vi "TB-Create Stimulus.vi"(0 "StimChan In":T24(xcontrol), 5 "state":T1, 11 "error in (no error)":errorcluster, 12 "Fine adjust (dB)":dbl) -> (4 "StimChan Out":T24(xcontrol), 6 "state out":T1, 8 "Stimulus":dbl[][](array[numeric]), 15 "error out":errorcluster)   [LabVIEW 2020]
uses:
  epl-vi-lib/Signal Synthesis VIs/Controls/Stimulus Channel XCtl/Stimulus Channel.xctl
  Typedefs/TB-Stimulus State.ctl
  <vilib>/sound2/lvsound2.llb/Sound File Refnum.ctl
  epl-vi-lib/Utility VIs/Math VIs/dB to Linear (scalar).vi
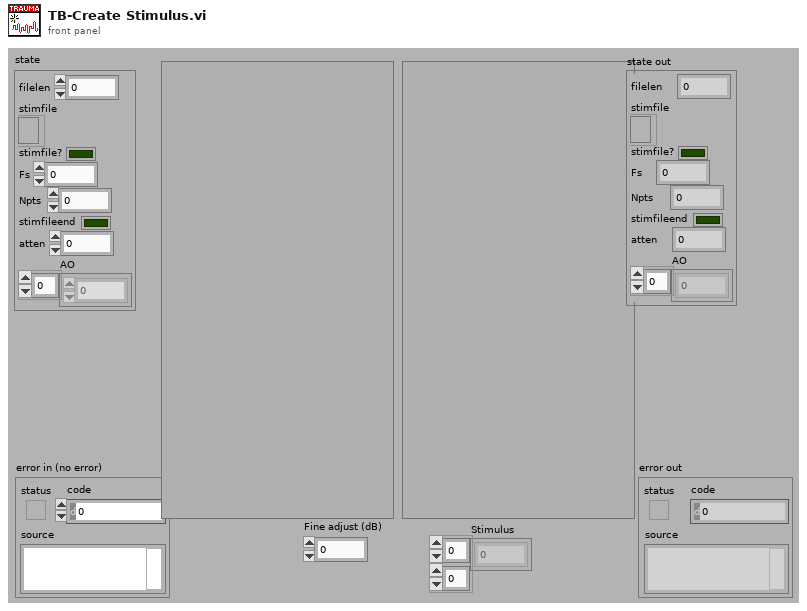
[diagram p1: front panel]
types:
  T1 = typedef "TB-Stimulus State.ctl" = cluster{"filelen":i32, "stimfile":T2, "stimfile?":bool, "Fs":dbl, "Npts":i32, "stimfileend":bool, "atten":dbl, "AO":i32[]}
  T2 = typedef "Sound File Refnum.ctl" = refnum<file>
  T3 = typedef "Waveform XCtl.xctl/Waveform Data.ctl" = cluster{"Type":T4, "Tone":T5, "Pulse Train":T6, "Noise":T9, "File":T10, "FMSweep":T11, "Chirp Train":T12, "Complex Tone":cluster{"Params":T14, "Data":T16}, "Moving Ripple":T17}
  T4 = typedef "Waveform Enum.ctl" = enum16{"OFF", "Tone", "Noise", "Pulse Train", "File", "FM Sweep", "Chirp Train", "Complex Tone", "FM Tone", "Moving Ripple"}
  T5 = typedef "Tone Params.ctl" = cluster{"Frequency (kHz)":dbl, "Last Freq":dbl, "Last Phase":dbl}
  T6 = typedef "Pulse Train Params.ctl" = cluster{"Pulse width (us)":dbl, "Pulse rate (Hz)":dbl, "Gap (ms)":dbl, "Polarity":T7, "PT State":T8, "Asynch":bool}
  T7 = typedef "Pulse Polarity.ctl" = enum16{"POS", "NEG", "POS-NEG", "NEG-POS"}
  T8 = typedef "PT-Continuous State.ctl" = cluster{"Template":dbl[], "Nperiod":i32, "Index":i32, "Pulse Rate (Hz)":dbl, "Phase (cycles)":dbl, "Noff":i32}
  T9 = typedef "Noise Params.ctl" = cluster{"InvFilt":bool, "Noise":dbl[], "CurPt":i32, "Aweight":bool, "Seed":i32, "afile":path}
  T10 = typedef "StimFile-Params.ctl" = cluster{"Filename":path, "Signal":dbl[], "Channel":i32, "stream":bool, "offset":i32, "nreps":i32, "loops":i32, "Randomize":bool, "order":i32[], "Seed":i32, "Tokens":i32}
  T11 = typedef "FM Sweep Params.ctl" = cluster{"Rate (oct/s)":dbl, "Fmin (Hz)":dbl, "Fmax (Hz)":dbl, "Ramp (ms)":dbl, "Linear":bool}
  T12 = typedef "Chirp Train.ctl" = cluster{"Params":T13, "Data":cluster{"WF":dbl[]}}
  T13 = typedef "Chirp Train Params.ctl" = cluster{"Fmin (kHz)":dbl, "Fmax (kHz)":dbl, "Compensate":bool, "Duration (ms)":dbl}
  T14 = typedef "CT-Params.ctl" = cluster{"F0 (Hz)":dbl, "Band":cluster{"Flow (Hz)":dbl, "Fhigh (Hz)":dbl}, "Phase":T15, "Min F0 (Hz)":dbl, "Max F0 (Hz)":dbl, "ContinRandPhase":bool, "Max peak factor":dbl, "Max mod depth":dbl, "MinHarmNum":i32, "MaxHarmNum":i32, "Level Mode":enum16{"per component", "overall rms"}, "% jitter":dbl}
  T15 = typedef "CT-Phase Enum.ctl" = enum16{"Cosine", "Random", "Alternating"}
  T16 = typedef "CT-Runtime Data.ctl" = cluster{"Ncomp":i32, "MinHarm":i32, "Phase":dbl[], "Amplitude":dbl[], "Npts/frame":i32, "Last F0":dbl, "Fmin":dbl, "Fmax":dbl, "Lslope":dbl, "randphase":bool, "overall rms":bool, "fmult":dbl[], "jittered":bool}
  T17 = typedef "Moving Ripple.ctl" = cluster{"Params":T18, "Data":T19}
  T18 = typedef "Moving Ripple.Params.ctl" = cluster{"Fmin":dbl, "Fmax":dbl, "Density":dbl, "Velocity":dbl, "Depth":dbl, "Phase":dbl, "Comp/oct":i32}
  T19 = typedef "Moving Ripple.Data.ctl" = cluster{"Freq":dbl[], "A":dbl[], "phase":dbl[], "Phase":dbl}
  T20 = typedef "Filter XCtl.xctl/Filter Data.ctl" = cluster{"CF (kHz)":dbl, "BW (kHz)":dbl, "IIR Filter Cluster":cluster{"filter structure":enum32{"IIR 2nd Order", "IIR 4th Order"}, "Reverse Coefficients":dbl[], "Forward Coefficients":dbl[]}, "Final Filter State":dbl[], "Scale Factor":dbl, "Final Filter State 2":dbl[], "Quadrature":bool, "Type":enum16{"Lowpass", "Highpass", "Bandpass", "Bandstop", "OFF"}}
  T21 = typedef "Gate Control.xctl/Gate Data.ctl" = cluster{"Active":bool, "Delay (ms)":dbl, "Width (ms)":dbl, "Ramp (ms)":dbl}
  T22 = typedef "Level XCtl.xctl/Level Data.ctl" = cluster{"Level":dbl, "Units":T23, "Max":dbl, "Multiplier":dbl, "Cal File":path, "Cal":cluster{"Freq (Hz)":dbl[], "Mag (dB SPL)":dbl[], "Phase (deg)":dbl[]}}
  T23 = typedef "Level Units.ctl" = enum16{"dB atten", "dB SPL", "dB re 1 Vrms", "dB V/Hz½", "mW", "dB HL", "Volts", "dB mW"}
  T24 = cluster{"Waveform":T3, "Filter":T20, "Gate":T21, "Level":T22}
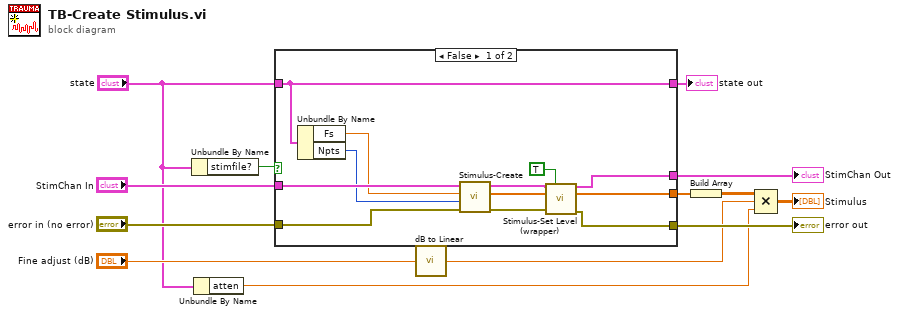
[diagram p0: block diagram]
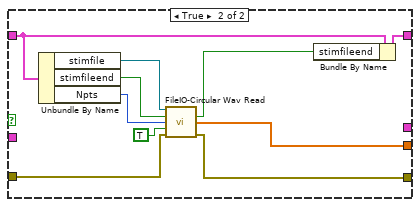
[diagram p2: hidden frame]
diagram:
  n1 = Unbundle By Name("state") -> ("stimfile?"=w4:bool)
  n2 = Unbundle By Name("state") -> ("atten"=w1:dbl)
  n3 = case shown="False" w4 {
    tunnel: "error in (no error)" -> [w25 w29]
    tunnel: "StimChan In" -> [w24 _]
    tunnel: [w19 _] -> w11
    tunnel: [w18 w27] -> w10
    tunnel: [w17 w28] -> w9
    tunnel: "state" -> [w14 w35]
    tunnel: [w14 w34] -> w3
    frame False {
      n4 = Unbundle By Name(w14) -> ("Fs"=w16:dbl, "Npts"=w15:i32)
      n5 = call "Stimulus-Create.vi"("error in (no error)"=w25, "Npts"=w15, "Sampling Rate (Hz)"=w16, "Stimulus Channel"=w24) -> ("error out"=w22:errorcluster, "Waveform"=w21:dbl[], "Stimulus Channel out"=w20:T24)  [unwired: 4 in, 1 out]
      n6 = call "Stimulus-Set Level (wrapper).vi"("Stimulus Channel"=w20, "Apply multiplier? (F)"=TRUE ("Apply multiplier?"), "Waveform in"=w21, "error in (no error)"=w22) -> ("Stimulus Channel out"=w19:T24, "Waveform out"=w18:dbl[], "error out"=w17:errorcluster)  [unwired: 7 in, 2 out]
    }
    frame True {
      n7 = Unbundle By Name(w35) -> ("stimfile"=w32:T2, "stimfileend"=w31:bool, "Npts"=w33:i32)
      n8 = call "FileIO-Circular Wav Read.vi"("Fileref in"=w32, "stimfileend"=w31, "Nread"=w33, "Loop?"=TRUE, "error in (no error)"=w29) -> ("end of file?"=w26:bool, "Y"=w27:dbl[], "error out"=w28:errorcluster)  [unwired: 6 in, 2 out]
      n9 = Bundle By Name(cluster=w35, "stimfileend"=w26) -> (w34:T1)
    }
  }
  "error out" <- w9
  "StimChan Out" <- w11
  "state out" <- w3
  n10 = call-poly "dB to Linear.vi"("dB"="Fine adjust (dB)") -> ("linear"=w5:dbl)
  n11 = Build Array(w10) -> (w8:dbl[][])
  n12 = Compound Arithmetic op=MULTIPLY(w8, w5, w1) -> (→"Stimulus":dbl[][])
